vi "Simulation_Current.vi"() -> ()   [LabVIEW 2015]
uses:
  <vilib>/Platform/TimedLoop/XDataNode/timing_clust.ctl
  <vilib>/Platform/TimedLoop/XDataNode/nitl_modes.ctl
  <vilib>/Platform/TimedLoop/XDataNode/wakeup.ctl
  <vilib>/Utility/file.llb/Read From Spreadsheet File (DBL).vi
  <vilib>/platform/TimedLoop/XDataNode/XDataNode.xnode
  <vilib>/Platform/TimedLoop/XDataNode/XDNodeRunTimeDep.lvlib
panel:
  in  "stop":bool
  out "element":dbl
  out "Waveform Chart":dbl(graph)
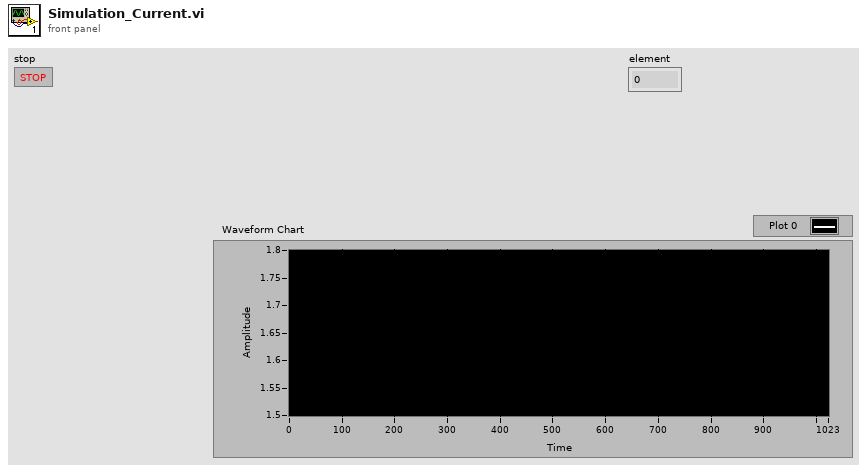
[diagram p1: front panel]
types:
  T1 = typedef "XDNodeRunTimeDep.lvlib/timing_clust.ctl" = cluster{"Expected End [f-1]":u64, "Actual End [f-1]":u64, "Finished Late? [f-1]":bool, "Expected End [i-1]":u64, "Actual End [i-1]":u64, "Finished Late? [i-1]":bool, "Expected Start [i]":u64, "Actual Start [i]":u64, "Expected Start [f]":u64, "Actual Start [f]":u64, "Source Name":string, "Structure Name":string, "Period":i64, "Deadline":i64, "Offset":i64, "Start":i64, "Priority":i32, "Timeout":i32, "Mode":T2, "Wakeup Reason":T3, "Error":errorcluster, "Source Type":string, "Secondary Source Type":string, "Global End Time":u64, "Global Start Time":u64, "Frame Duration":u64, "Iteration Duration":u64, "Assigned CPU":i32, "I/O Scan Engine Mode":u32}
  T2 = typedef "XDNodeRunTimeDep.lvlib/nitl_modes.ctl" = enum32{"No Change", "Process missed periods, maintain original phase", "Discard missed periods, maintain original phase", "Process missed periods, ignore original phase", "Discard missed periods, ignore original phase"}
  T3 = typedef "XDNodeRunTimeDep.lvlib/wakeup.ctl" = enum32{"Normal", "Aborted", "Asynchronous wakeup", "Timing source error", "Timed loop error", "Timeout"}
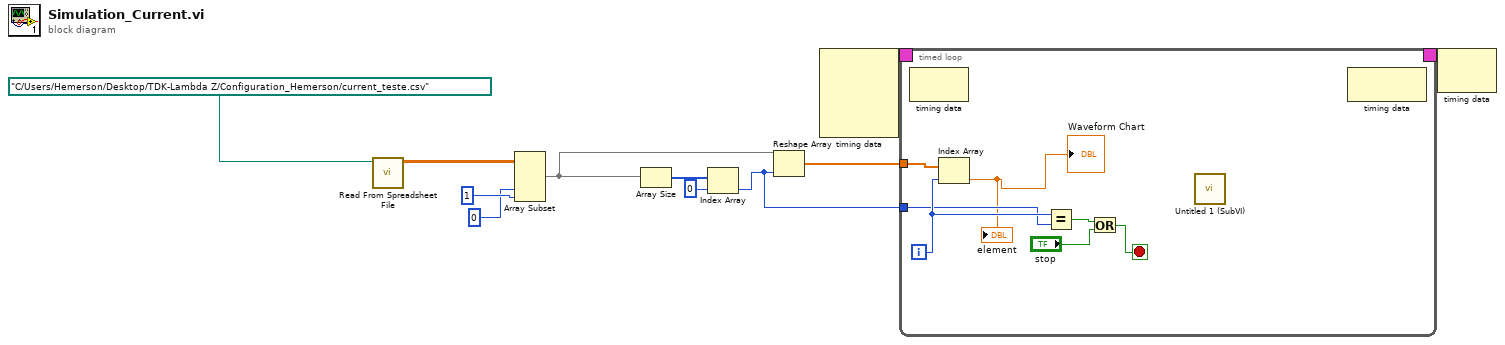
[diagram p0: block diagram]
diagram:
  n1 = call-poly <vilib>:"Read From Spreadsheet File.vi"("file path (dialog if empty)"=path "C:/Users/Hemerson/Desktop/TDK-Lambda Z/Configuration_Hemerson/current_teste.csv") -> ("all rows"=w7:dbl[][])  [unwired: 6 in, 4 out]
  n2 = Array Subset "Array Subset"(array=w7, index (col)=0 ("index"), length (col)=1 ("length")) -> (w2:dbl[][])  [unwired: 2 in]
  n3 = Array Size(array=w2) -> (size(s)=w9:i32[])
  n4 = Index Array "Index Array"(array=w9, index=0) -> (element=w1:i32)
  n5 = Reshape Array "Reshape Array"(w2, w1) -> (w3:dbl[])
  n6 = node-c288() -> (w5:T1)  [unwired: 4 in]
  n7 = timed-loop {
    timing: w5 -> [_]
    timing-out: [_] -> w4
    tunnel: w3 -> [w13]
    tunnel: w1 -> [w17]
    i -> [w18]
    stop <- w16 stop-if-true
    n8 = node-c288() -> ()  [unwired: 1 in, 1 out]
    n9 = Index Array(array=w13, index=w18) -> (element=→"element" →"Waveform Chart":dbl)
    n10 = Equal?(x=w18, y=w17) -> (x = y?=w15:bool)
    n11 = Or(x=w15, y="stop") -> (x .or. y?=w16:bool)
    n12 = call "Untitled 1 (SubVI).vi"() -> ()  [unwired: 13 in, 7 out]
    n13 = node-c288() -> ()  [unwired: 1 in, 1 out]
  }
  n14 = node-c288(w4) -> ()  [unwired: 1 out]
